vi "Abort Channel.vi"(8 "sync in":errorcluster) -> (2 "channel":T1)   [LabVIEW 2020, in "Cmd-Data Event Messages.lvlib"]
doc: "Aborts the channel connected to this VI. This VI executes normally even if there is an error at sync in."
uses:
  Cmd-Data Event Messages.lvlib
  <extravilib>/ChannelInstances/Event Messenger Priority-c(str,var).lvlib
  <extravilib>/ChannelInstances/Event Messenger Priority-c(str,var)/))Channel.ctl
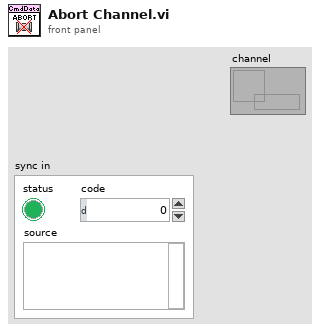
[diagram p1: front panel]
types:
  T1 = typedef "Event Messenger Priority-c(str,var).lvlib/))Channel.ctl" = refnum<queue>
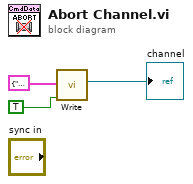
[diagram p0: block diagram]
diagram:
  n1 = call <extravilib>:"Write.vi"("abort (F)"=TRUE, "element"=cluster{"cmd":string, "data":variant} {"cmd"="", "data"=variant}) -> ("channel"=→"channel":T1)  [unwired: 8 in, 1 out]
